vi "_RT_CtrlLoop_Log stateMachine.vi"(8 "error in (no error)":errorcluster, 11 "RTLogQueue in":refnum<queue>) -> (0 "error out":errorcluster)   [LabVIEW 2018]
uses:
  <vilib>/Platform/TimedLoop/XDataNode/timing_clust.ctl
  <vilib>/Platform/TimedLoop/XDataNode/nitl_modes.ctl
  <vilib>/Platform/TimedLoop/XDataNode/wakeup.ctl
  <vilib>/Platform/TimedLoop/XDataNode/XDataNode.xnode
  <vilib>/Platform/TimedLoop/XDataNode/XDNodeRunTimeDep.lvlib
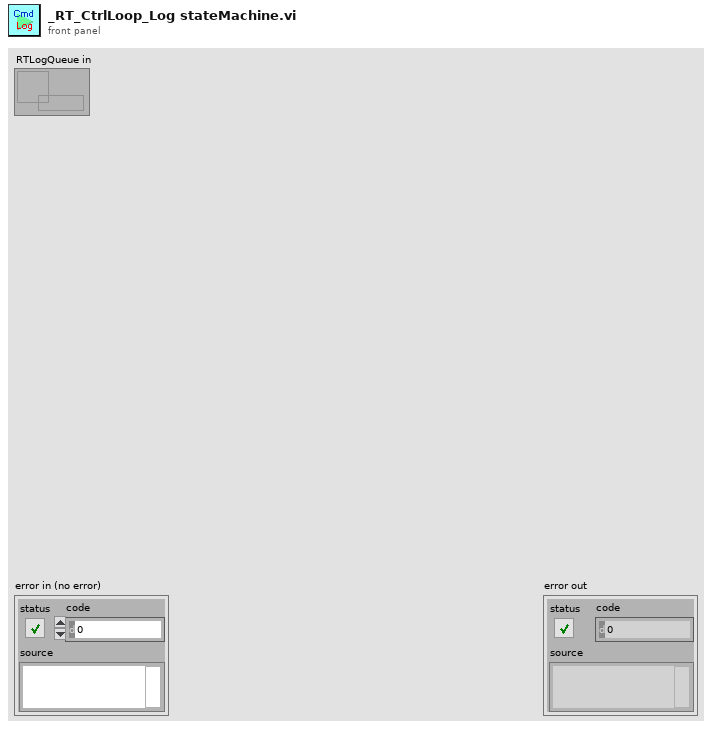
[diagram p1: front panel]
types:
  T1 = typedef "XDNodeRunTimeDep.lvlib/timing_clust.ctl" = cluster{"Expected End [f-1]":u64, "Actual End [f-1]":u64, "Finished Late? [f-1]":bool, "Expected End [i-1]":u64, "Actual End [i-1]":u64, "Finished Late? [i-1]":bool, "Expected Start [i]":u64, "Actual Start [i]":u64, "Expected Start [f]":u64, "Actual Start [f]":u64, "Source Name":string, "Structure Name":string, "Period":i64, "Deadline":i64, "Offset":i64, "Start":i64, "Priority":i32, "Timeout":i32, "Mode":T2, "Wakeup Reason":T3, "Error":errorcluster, "Source Type":string, "Secondary Source Type":string, "Global End Time":u64, "Global Start Time":u64, "Frame Duration":u64, "Iteration Duration":u64, "Assigned CPU":i32, "I/O Scan Engine Mode":u32}
  T2 = typedef "XDNodeRunTimeDep.lvlib/nitl_modes.ctl" = enum32{"No Change", "Process missed periods, maintain original phase", "Discard missed periods, maintain original phase", "Process missed periods, ignore original phase", "Discard missed periods, ignore original phase"}
  T3 = typedef "XDNodeRunTimeDep.lvlib/wakeup.ctl" = enum32{"Normal", "Aborted", "Asynchronous wakeup", "Timing source error", "Timed loop error", "Timeout"}
  T4 = cluster{"function type":enum16{"none", "init", "write", "read"}, "actionCmd":string, "callChain":string, "customErrorMsg":string, "error constant":errorcluster}
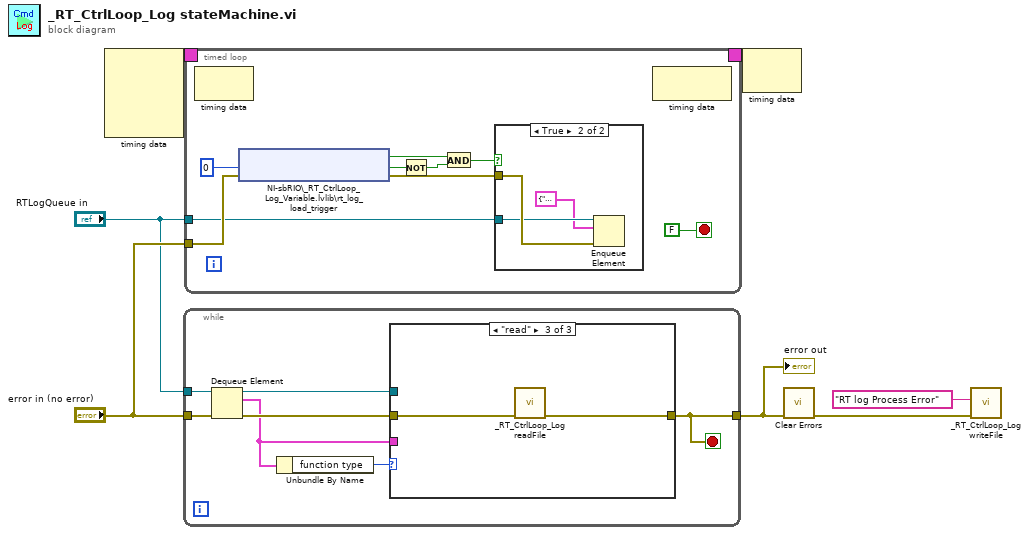
[diagram p0: block diagram]
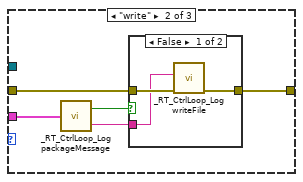
[diagram p3: hidden frame]
diagram:
  n1 = node-c288() -> (w7:T1)  [unwired: 4 in]
  n2 = while {
    tunnel: "RTLogQueue in" -> [w14]
    tunnel: "error in (no error)" -> [w13]
    tunnel: [w8] -> w2
    stop <- w8 stop-if-true
    n3 = Dequeue Element(queue=w14, error in (no error)=w13) -> (queue out=w10:refnum<queue>, element=w9:T4, error out=w11:errorcluster)  [unwired: 1 in, 1 out]
    n4 = Unbundle By Name(w9) -> ("function type"=w12:enum16{"none", "init", "write", "read"})
    n5 = case shown="\"read\"" w12 {
      tunnel: w11 -> [w15 w20 w26]
      tunnel: w10 -> [_ _ _]
      tunnel: w9 -> [_ w18 _]
      tunnel: [w15 w19 w25] -> w8
      frame "none", Default {
      }
      frame "write" {
        n6 = call "_RT_CtrlLoop_Log packageMessage.vi"("logCluster"=w18) -> ("igore"=w16:bool, "Message"=w17:string)
        n7 = case shown="False" w16 {
          tunnel: w20 -> [w23 w24]
          tunnel: [w22 w24] -> w19
          tunnel: w17 -> [w21 _]
          frame False {
            n8 = call "_RT_CtrlLoop_Log writeFile.vi"("error in"=w23, "Describe"=w21) -> ("error out"=w22:errorcluster)  [unwired: 9 in]
          }
          frame True {
          }
        }
      }
      frame "read" {
        n9 = call "_RT_CtrlLoop_Log readFile.vi"("error in"=w26) -> ("error out"=w25:errorcluster)  [unwired: 10 in]
      }
    }
  }
  "error out" <- w2
  n10 = timed-loop {
    timing: w7 -> [_]
    timing-out: [_] -> w6
    tunnel: "RTLogQueue in" -> [w32]
    tunnel: "error in (no error)" -> [w33]
    stop <- FALSE stop-if-true
    n11 = node-c288() -> ()  [unwired: 1 in, 1 out]
    n12 = shared-variable "NI-sbRIO\\_RT_CtrlLoop_Log_Variable.lvlib\\rt_log_load_trigger"(error in=w33, 0 ("ms timeout (0)")) -> (w29:bool, error out=w34:errorcluster, w30:bool)
    n13 = Not(x=w30) -> (.not. x?=w28:bool)
    n14 = And(x=w29, y=w28) -> (x .and. y?=w27:bool)
    n15 = case shown="True" w27 {
      tunnel: w34 -> [_ w38]
      tunnel: w32 -> [_ w37]
      frame False {
      }
      frame True {
        n16 = Enqueue Element(queue=w37, element=T4 {"function type"=enum."read", "actionCmd"="", "callChain"="", "customErrorMsg"="", "error constant"={"status"=FALSE, "code"=0, "source"=""}}, error in (no error)=w38) -> ()  [unwired: 1 in, 3 out]
      }
    }
    n17 = node-c288() -> ()  [unwired: 1 in, 1 out]
  }
  n18 = node-c288(w6) -> ()  [unwired: 1 out]
  n19 = call <vilib>:"Clear Errors.vi"("error in (no error)"=w2) -> ("error out"=w3:errorcluster)  [unwired: 5 in, 1 out]
  n20 = call "_RT_CtrlLoop_Log writeFile.vi"("error in"=w3, "Describe"="RT log Process Error") -> ()  [unwired: 9 in, 1 out]
